vi "Read EXE Path.vi"(8 "error in (no error)":errorcluster, 11 "CallEXEStep in":refnum<class "CallEXEStep.lvclass">) -> (0 "error out":errorcluster, 2 "EXE Path":string, 3 "CallEXEStep out":refnum<class "CallEXEStep.lvclass">)   [LabVIEW 2015, in "CallEXEStep.lvclass"]
uses:
  CallEXEStep.lvclass
  CallEXEStep.lvclass/CallEXEStep.ctl
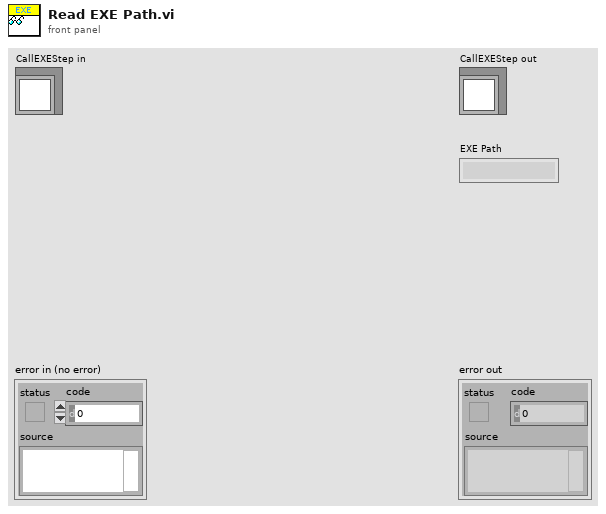
[diagram p1: front panel]
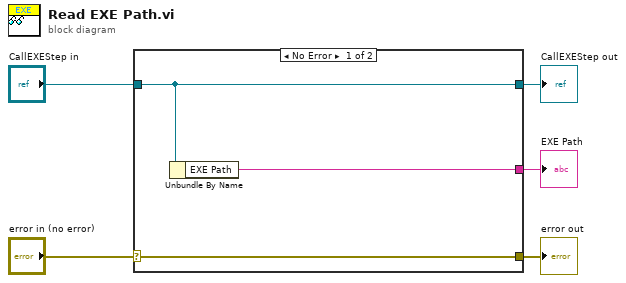
[diagram p0: block diagram]
diagram:
  n1 = case shown="No Error" "error in (no error)" {
    selector: "error in (no error)" -> [w8 w9]
    tunnel: [w8 w9] -> w4
    tunnel: [w7 w10] -> w2
    tunnel: "CallEXEStep in" -> [w7 w10]
    tunnel: [w6 _] -> w1
    frame No Error {
      n2 = Unbundle By Name(w7) -> ("EXE Path"=w6:string)
    }
    frame Error {
    }
  }
  "error out" <- w4
  "CallEXEStep out" <- w2
  "EXE Path" <- w1
